vi "Check if Click in Graph Legend.vi"(8 "error in (no error)":errorcluster, 10 "Mouse Coords":T1, 11 "WaveformGraph":refnum<vi>) -> (0 "error out":errorcluster, 2 "click in legend?":bool)   [LabVIEW 2021, in "Single Tone_Class D Amplifier_UI.lvlib"]
uses:
  Single Tone_Class D Amplifier_UI.lvlib
  <vilib>/Utility/miscctls.llb/LVPoint32TypeDef.ctl
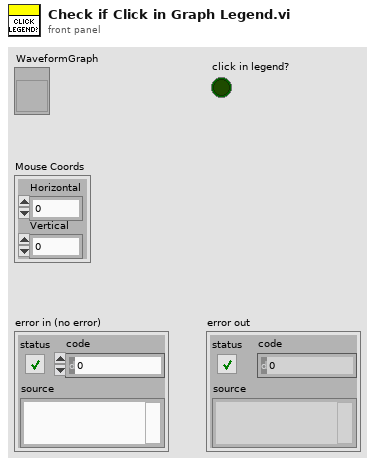
[diagram p1: front panel]
types:
  T1 = typedef "LVPoint32TypeDef.ctl" = cluster{"Horizontal":i32, "Vertical":i32}
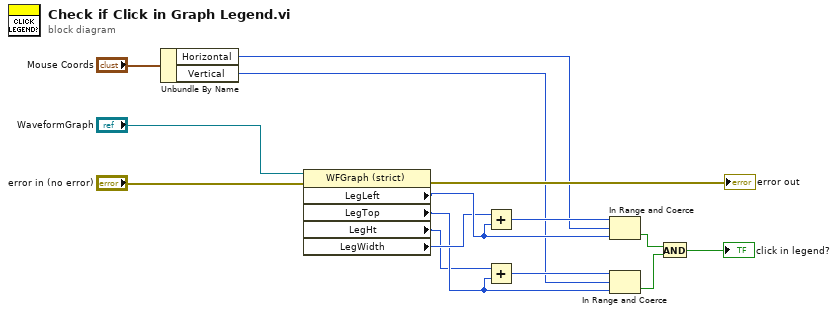
[diagram p0: block diagram]
diagram:
  n1 = Unbundle By Name("Mouse Coords") -> ("Horizontal"=w5:i32, "Vertical"=w4:i32)
  n2 = property class="WFGraph (strict)"(reference="WaveformGraph", error in="error in (no error)") -> (error out=→"error out":errorcluster, "LegLeft"=w10:i32, "LegTop"=w8:i32, "LegHt"=w7:u32, "LegWidth"=w9:u32)  [unwired: 1 out]
  n3 = Add(x=w9, y=w10) -> (x+y=w12:u32)
  n4 = Add(x=w7, y=w8) -> (x+y=w11:u32)
  n5 = In Range and Coerce(upper limit=w12, x=w5, lower limit=w10) -> (In Range?=w3:bool)  [unwired: 1 out]
  n6 = In Range and Coerce(upper limit=w11, x=w4, lower limit=w8) -> (In Range?=w2:bool)  [unwired: 1 out]
  n7 = And(x=w3, y=w2) -> (x .and. y?=→"click in legend?":bool)
